vi "Get real whale.vi"(2 "error in":errorcluster, 3 "Image":T2) -> (0 "error out":errorcluster, 1 "Matches":T1(array[cluster]) {"Bounding Box"."y" format="%.2f"; "Bounding Box"."x" format="%.2f"; "Position"."y" format="%.2f"; "Position"."x" format="%.2f"; "Score" format="%.2f"; "Scale" format="%.2f"; "Angle" format="%.2f"})   [LabVIEW 2011]
uses:
  <vilib>/vision/Image Controls.llb/IMAQ Image.ctl
panel:
  out "Templete Image":T2(plugin-control)
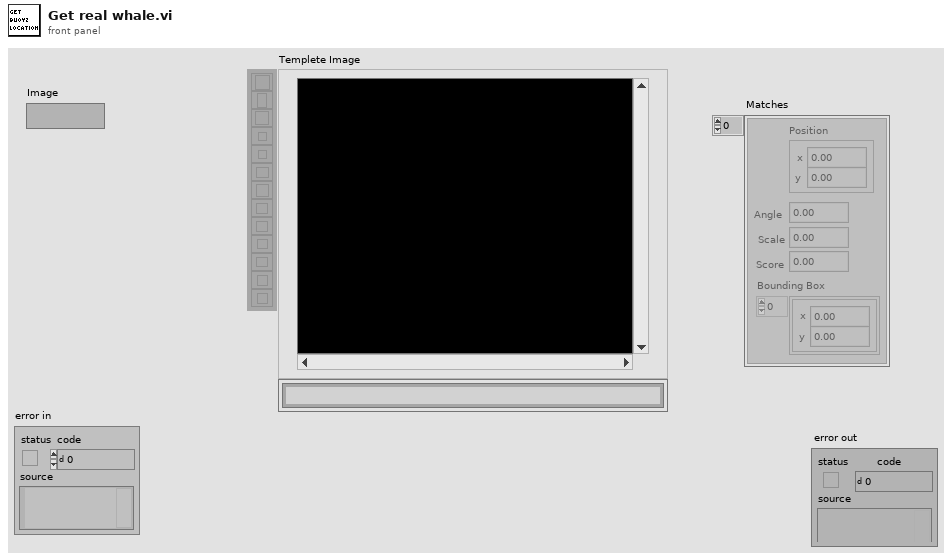
[diagram p1: front panel]
types:
  T1 = cluster{"Position":cluster{"x":sgl, "y":sgl}, "Angle":sgl, "Scale":sgl, "Score":sgl, "Bounding Box":cluster{"x":sgl, "y":sgl}[]}[]
  T2 = typedef "IMAQ Image.ctl" = refnum<image>
  T3 = cluster{"Global Rectangle":i32[], "Contours":cluster{"ID":enum32{"External", "Internal"}, "Type":u32, "Coordinates":i32[]}[]}
  T4 = typedef "Image Type" = u32
  T5 = cluster{"Match Mode (Pattern Matching 1)":u16, "Subpixel Accuracy (Pattern Matching 1)":bool, "Rotation Angle Ranges (degrees) (Pattern Matching 1)":cluster{sgl, sgl}[]}
  T6 = cluster{"ROI Descriptor (Geometric Matching 1)":cluster{"Global Rectangle":i32[], "Contours":cluster{"ID":enum32{"External", "Internal"}, "Type":u32, "Coordinates":i32[]}[]}, "Number of Matches Requested (Pattern Matching 1)":i32, "Minimum Match Score (Pattern Matching 1)":sgl}
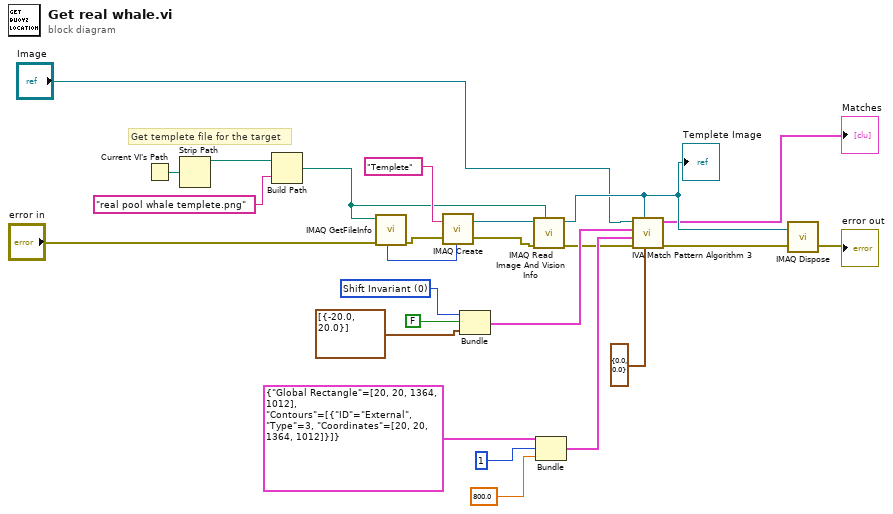
[diagram p0: block diagram]
diagram:
  w14 = u16 0 items=["Shift Invariant", "Rotation Invariant"] ("Match Mode (Pattern Matching 1)")
  # "Get templete file for the target"
  n1 = Current VI's Path() -> (path=w23:path)
  n2 = Strip Path(path=w23) -> (stripped path=w22:path)  [unwired: 1 out]
  n3 = Build Path(base path=w22, name or relative path="real pool whale templete.png") -> (appended path=w18:path)
  n4 = call "IMAQ GetFileInfo"("error in (no error)"="error in", "File Path"=w18) -> ("error out"=w21:errorcluster, "Image Type"=w20:T4)  [unwired: 3 in, 5 out]
  n5 = call "IMAQ Create"("Image Name"="Templete", "Image Type"=w20, "error in (no error)"=w21) -> ("New Image"=w16:T2, "error out"=w17:errorcluster)  [unwired: 1 in, 1 out]
  n6 = Bundle("Match Mode (Pattern Matching 1)"=w14, "Subpixel Accuracy (Pattern Matching 1)"=FALSE, "Rotation Angle Ranges (degrees) (Pattern Matching 1)"=cluster{sgl, sgl}[] [{-20.0, 20.0}]) -> (w6:T5)  [unwired: 1 out]
  n7 = call "IMAQ Read Image And Vision Info"("File Path"=w18, "error in (no error)"=w17, "Image"=w16) -> ("error out"=w3:errorcluster, "Image Out"=w9:T2)  [unwired: 1 in, 6 out]
  "Templete Image" <- w9
  n8 = Bundle("ROI Descriptor (Geometric Matching 1)"=T3 {"Global Rectangle"=[20, 20, 1364, 1012], "Contours"=[{"ID"=enum."External", "Type"=3, "Coordinates"=[20, 20, 1364, 1012]}]}, "Number of Matches Requested (Pattern Matching 1)"=1, "Minimum Match Score (Pattern Matching 1)"=sgl 800.0) -> (w5:T6)  [unwired: 1 out]
  n9 = call <vilib>:"IVA Match Pattern Algorithm 3.vi"("Match Offset"=cluster{"X":sgl, "Y":sgl} {"X"=0.0, "Y"=0.0} ("Match Offset (Pattern Matching 1)"), "Image Template"=w9, "error in (no error)"=w3, "Match Parameters"=w5, "Setup Match Parameters"=w6, "Image"="Image") -> ("error out"=w2:errorcluster, "Matches"=→"Matches":T1)  [unwired: 4 out]
  n10 = call "IMAQ Dispose"("Image"=w9, "error in (no error)"=w2) -> ("error out"=→"error out":errorcluster)  [unwired: 4 in]
